vi "SetStrArrTo1DArrayCtrl.vi"(10 "str arr":string[](array[string]), 11 "array in":refnum<vi>) -> ()   [LabVIEW 2018, in "Library-Ctrl.lvlib"]
uses:
  Library-Ctrl.lvlib
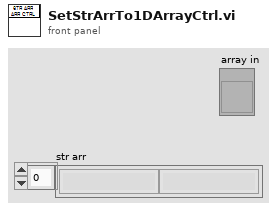
[diagram p1: front panel]
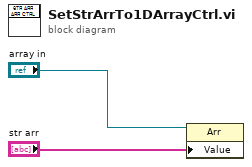
[diagram p0: block diagram]
diagram:
  n1 = property class="Arr"(reference="array in", "Value"="str arr") -> ()  [unwired: 1 in, 2 out]
